vi "String - String to EditPos Cluster.vi"(11 "string":string) -> (3 "EditPos":cluster{"row":i32, "col":i32})   [LabVIEW 2013]
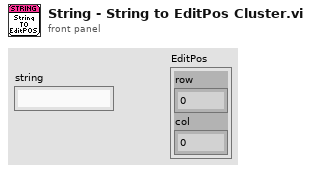
[diagram p1: front panel]
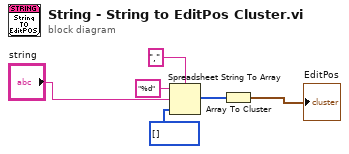
[diagram p0: block diagram]
diagram:
  n1 = Spreadsheet String To Array(delimiter (Tab)=",", format string="%d", spreadsheet string="string", array type (2D Dbl)=i32[] []) -> (array=w4:i32[])
  n2 = Array To Cluster(array=w4) -> (cluster=→"EditPos":cluster{"[0]":i32, "[1]":i32})
